vi "自动升级程序.vi"(8 "错误输入（无错误）":errorcluster) -> (0 "错误输出":errorcluster, 3 "确定":bool)   [LabVIEW 2016, in "数据传输系统.lvlib"]
uses:
  <vilib>/Utility/miscctls.llb/LVPointTypeDef.ctl
panel:
  in  "滚动条":i32(c297)
  out "标题":string
  in  "取消":bool
  in  "确定":bool
  out "版本说明显示":string
  # "是否立即下载新版本(download right now)?"
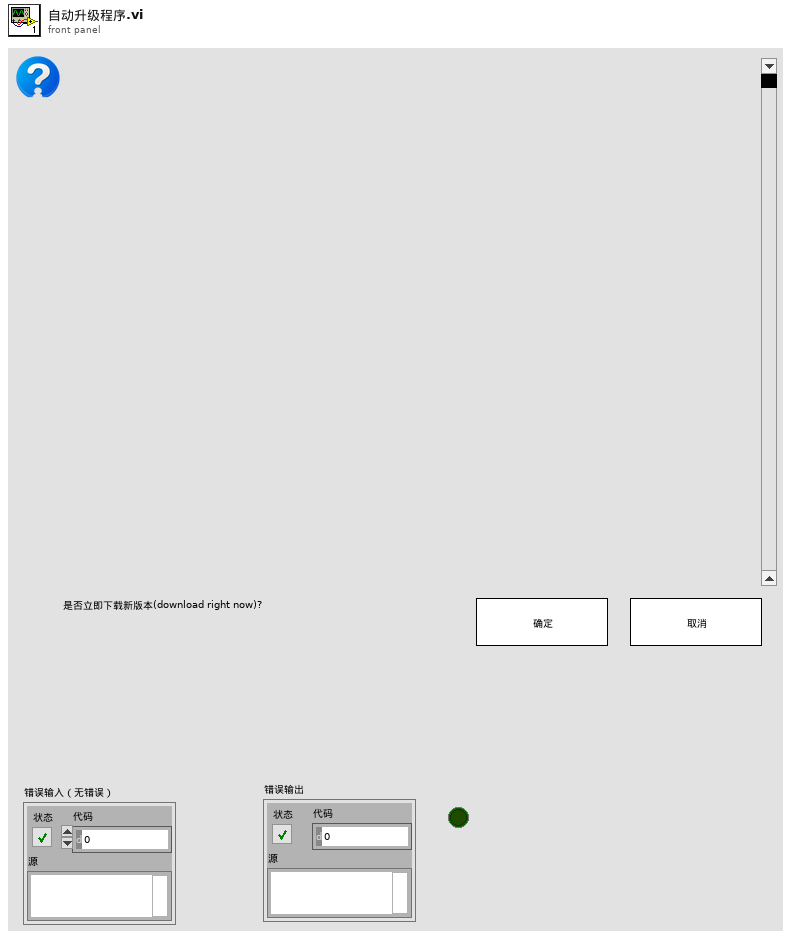
[diagram p1: front panel]
types:
  T1 = typedef "LVPointTypeDef.ctl" = cluster{"Horizontal":i16, "Vertical":i16}
  T2 = enum16{"open", "replace", "create", "open or create", "replace or create", "replace or create with confirmation"}
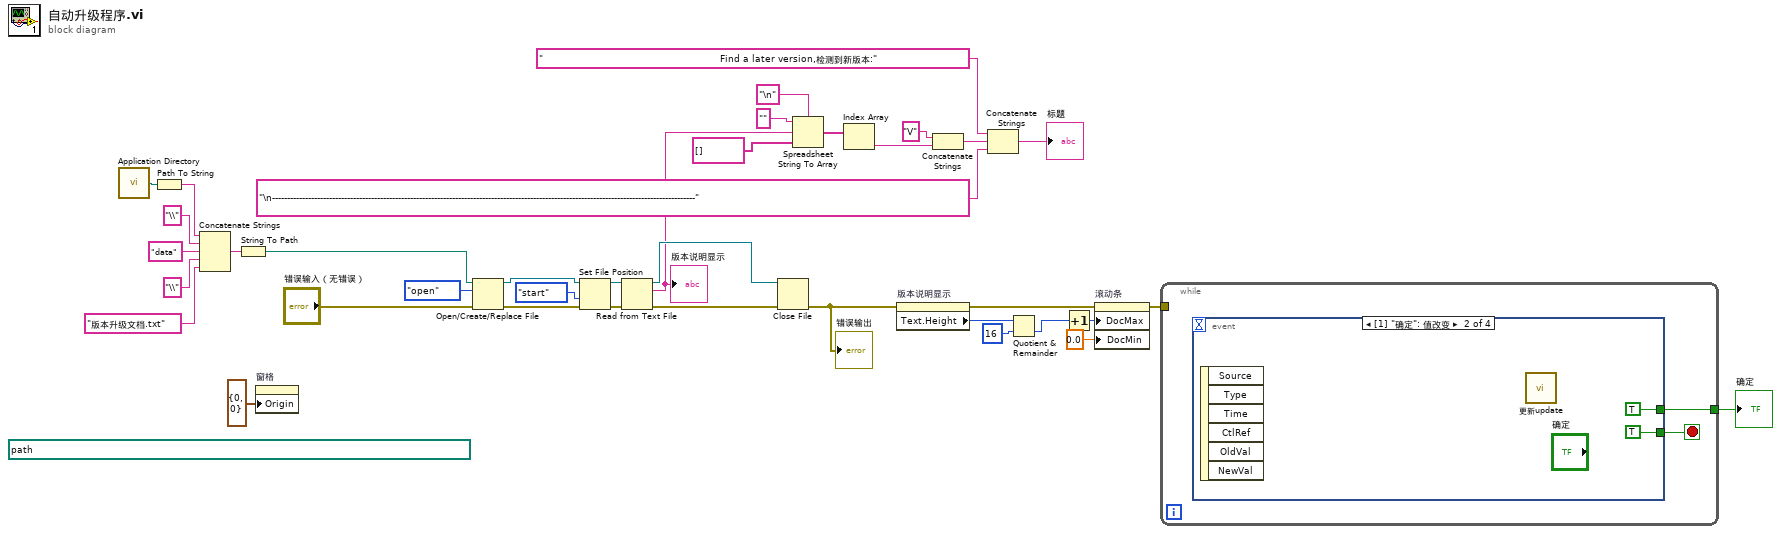
[diagram p0: block diagram]
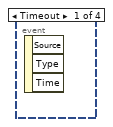
[diagram p2: hidden frame]
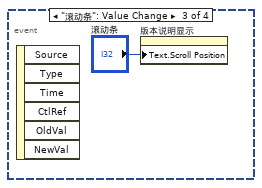
[diagram p3: hidden frame]
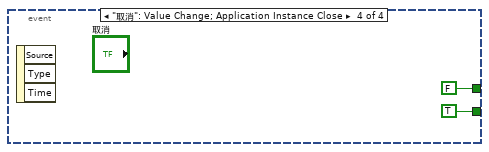
[diagram p4: hidden frame]
diagram:
  (unwired) path "F:/gitkraken/CC/平台数采程序 - V2.0.1（正式修改迭代版）/data/版本升级文档.txt" ("路径")
  n1 = call <vilib>:"Application Directory.vi"() -> ("Application Directory"=w26:path)
  n2 = Path To String(path=w26) -> (string=w29:string)
  n3 = Concatenate Strings(w29, "\\" ("字符串"), "data" ("字符串"), "\\" ("字符串"), "版本升级文档.txt" ("字符串")) -> (w23:string)
  n4 = String To Path(string=w23) -> (path=w2:path)
  n5 = property on="窗格" class="Pane"("Origin"=T1 {"Horizontal"=0, "Vertical"=0} ("原点")) -> ()  [unwired: 2 in, 2 out]
  n6 = Open/Create/Replace File(file path (use dialog)=w2, error in="错误输入（无错误）", operation (0:open)=T2."open" ("操作(0:open)")) -> (refnum out=w34:refnum<file>, error out=w33:errorcluster)  [unwired: 3 in, 1 out]
  n7 = Set File Position(refnum=w34, from (0:start)=enum16{"start", "end", "current"}."start" ("自（0:起始）"), error in=w33) -> (refnum out=w30:refnum<file>, error out=w32:errorcluster)  [unwired: 1 in]
  n8 = Read from Text File(file (use dialog)=w30, error in=w32) -> (refnum out=w36:refnum<file>, text=w18:string, error out=w37:errorcluster)  [unwired: 2 in, 1 out]
  "版本说明显示" <- w18
  n9 = Close File(refnum=w36, error in=w37) -> (error out=w4:errorcluster)  [unwired: 1 out]
  "错误输出" <- w4
  n10 = Spreadsheet String To Array(delimiter (Tab)="\n" ("分隔符(Tab)"), format string="" ("格式字符串"), spreadsheet string=w18, array type (2D Dbl)=string[] []) -> (array=w14:string[])
  n11 = Index Array(array=w14) -> (element=w13:string)  [unwired: 1 in]
  n12 = property on="版本说明显示" class="Str"(error in=w4) -> (error out=w5:errorcluster, "Text.Height"=w10:u32)  [unwired: 1 in, 1 out]
  n13 = Concatenate Strings("V" ("字符串"), w13) -> (w11:string)
  n14 = Concatenate Strings("                                                           Find a later version,检测到新版本:" ("标题"), w11, "\n---------------------------------------------------------------------------------------------------------------------------------------------" ("标题")) -> (→"标题":string)
  n15 = Quotient & Remainder(x=w10, y=u32 16) -> (floor(x/y)=w8:u32)  [unwired: 1 out]
  n16 = Increment(x=w8) -> (x+1=w3:u32)
  n17 = property on="滚动条" class="Scroll (严格)"(error in=w5, "DocMax"=w3, "DocMin"=0.0 ("滚动范围最小值")) -> (error out=w6:errorcluster)  [unwired: 1 in, 1 out]
  n18 = while {
    tunnel: [w39] -> w22
    tunnel: w6 -> [_]
    stop <- w40 stop-if-true
    n19 = event shown="[1] \"确定\": 值改变" {
      selector: _ -> [_ _ _ _]
      dyn-events: _ -> [_ _ _ _]
      timeout: _ -> [_ _ _ _]
      tunnel: [_ TRUE _ TRUE] -> w40
      tunnel: [_ TRUE ("确定") _ FALSE ("确定")] -> w39
      event Timeout {
        n20 = event-data() -> ()  [unwired: 1 in, 3 out]
      }
      event "确定": Value Change {
        n21 = event-data() -> ()  [unwired: 1 in, 6 out]
        n22 = call "更新update.vi"() -> ()  [unwired: 12 in]
      }
      event "滚动条": Value Change {
        n23 = event-data() -> ()  [unwired: 1 in, 6 out]
        n24 = property on="版本说明显示" class="Str"("Text.Scroll Position"="滚动条") -> ()  [unwired: 2 in, 2 out]
      }
      event "取消": Value Change; Application Instance Close {
        n25 = event-data() -> ()  [unwired: 1 in, 3 out]
      }
    }
  }
  "确定" <- w22
